vi "Node - Config Writer.vi"(8 "error in (no error)":errorcluster, 11 "Node Data In":T1) -> (0 "error out":errorcluster, 3 "Node Data Out":T1)   [LabVIEW 2016, in "PXImc Router.lvlib"]
uses:
  PXImc Router.lvlib
  Controls/Node Data.ctl
  <vilib>/NI Veristand/VeriStand Data/Byte Buffer/Byte Buffer.lvclass
  Controls/Node/Node - PXImc Parameters.ctl
  Controls/Node/Node - Writer Data.ctl
  Controls/Node/Node Ch Properties.ctl
  Controls/Data Type.ctl
  Controls/Node/Node - Readers Data.ctl
  Controls/Node/Node - Reader Data.ctl
  <vilib>/NI Veristand/VeriStand Data/Byte Buffer/Byte Buffer.lvclass/Byte Buffer.ctl
  <vilib>/NI Veristand/VeriStand Data/Byte Buffer/Byte Buffer.Get Buffer Pointer.vi
  <vilib>/NI Veristand/VeriStand Data/Byte Buffer/Byte Buffer.Get Buffer Size.vi
  <vilib>/NI Veristand/VeriStand Data/Memory Management/Memory Management.MoveByteBlock (Pointer).vi
  <vilib>/NI Veristand/VeriStand Data/Pointer Operations/Pointer.New.vi
  <vilib>/NI Veristand/VeriStand Data/Pointer Operations/Pointer.Dispose.vi
  <vilib>/NI Veristand/VeriStand Data/Byte Buffer/Byte Buffer.Set Buffer Pointer.vi
  <vilib>/NI Veristand/VeriStand Data/Byte Buffer/Byte Buffer.Set Buffer Size.vi
  <vilib>/NI Veristand/VeriStand Data/Memory Management/Memory Management.Handle Return.vi
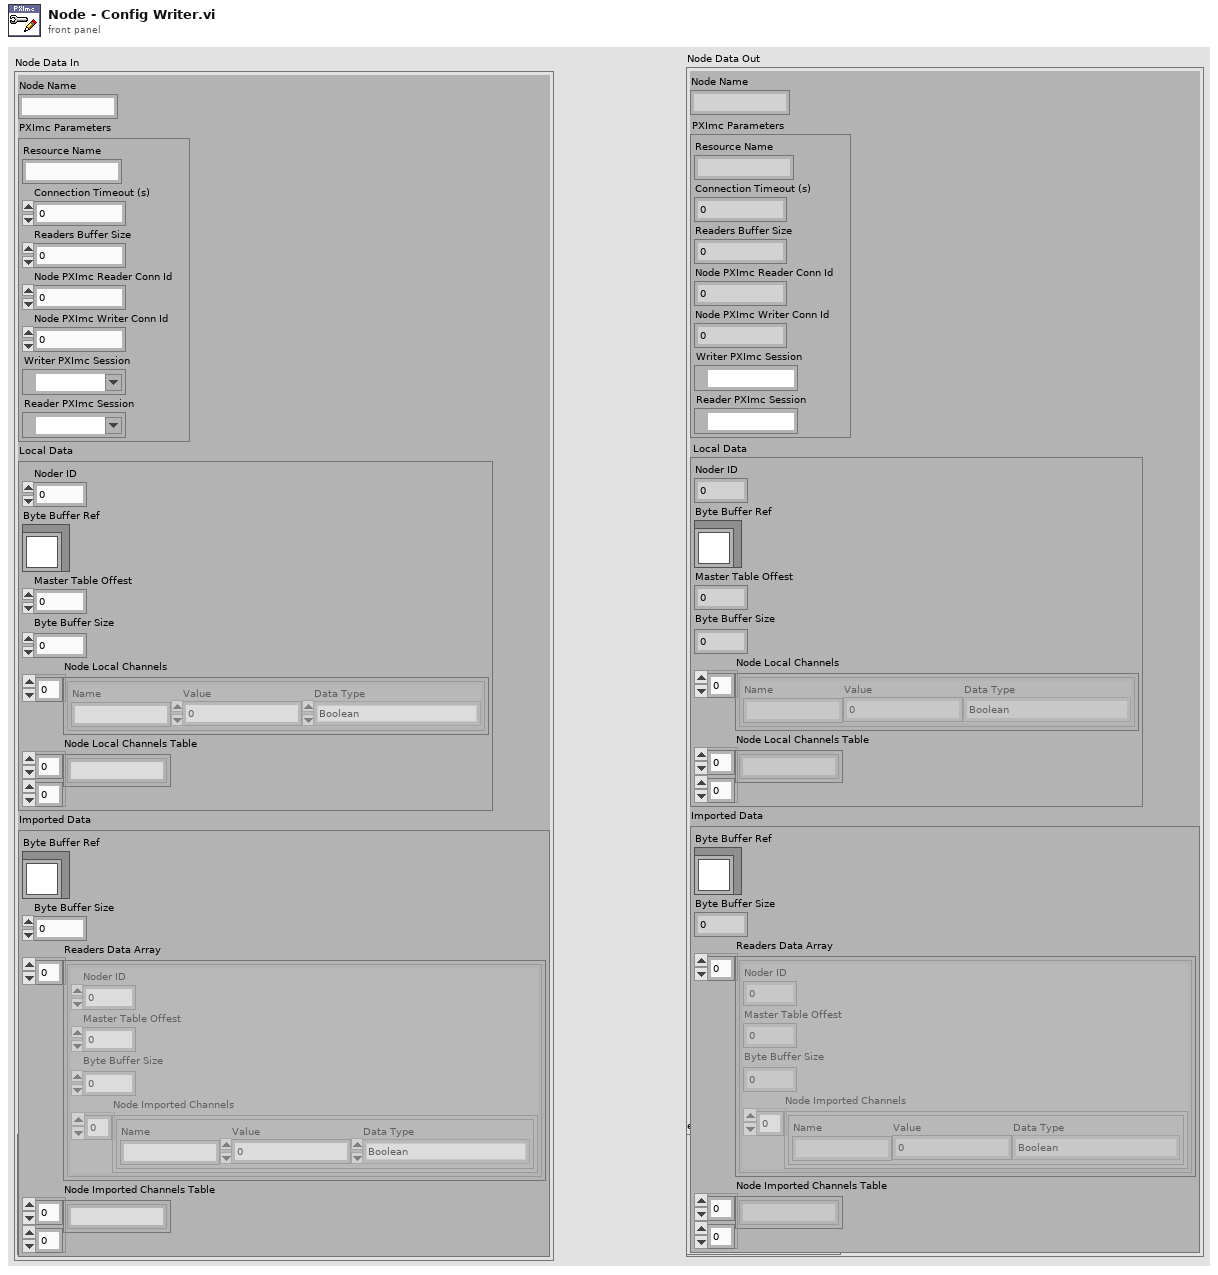
[diagram p1: front panel]
types:
  T1 = typedef "PXImc Router.lvlib/Node Data.ctl" = cluster{"Node Name":string, "PXImc Parameters":T2, "Local Data":T3, "Imported Data":T6}
  T2 = typedef "PXImc Router.lvlib/Node - PXImc Parameters.ctl" = cluster{"Resource Name":string, "Connection Timeout (s)":dbl, "Readers Buffer Size":u64, "Node PXImc Reader Conn Id":u16, "Node PXImc Writer Conn Id":u16, "Writer PXImc Session":refnum<k21>, "Reader PXImc Session":refnum<k21>}
  T3 = typedef "PXImc Router.lvlib/Node - Writer Data.ctl" = cluster{"Noder ID":u32, "Byte Buffer Ref":refnum<class "Byte Buffer.lvclass">, "Master Table Offest":u32, "Byte Buffer Size":u32, "Node Local Channels":T4[], "Node Local Channels Table":string[][]}
  T4 = typedef "PXImc Router.lvlib/Node Ch Properties.ctl" = cluster{"Name":string, "Value":dbl, "Data Type":T5}
  T5 = typedef "PXImc Router.lvlib/Data Type.ctl" = enum16{"Boolean", "SGL", "DBL", "I8", "I16", "I32", "I64", "U8", "U16", "U32", "U64"}
  T6 = typedef "PXImc Router.lvlib/Node - Readers Data.ctl" = cluster{"Byte Buffer Ref":refnum<class "Byte Buffer.lvclass">, "Byte Buffer Size":u64, "Readers Data Array":T7[], "Node Imported Channels Table":string[][]}
  T7 = typedef "PXImc Router.lvlib/Node - Reader Data.ctl" = cluster{"Noder ID":u32, "Master Table Offest":u32, "Byte Buffer Size":u64, "Node Imported Channels":T4[]}
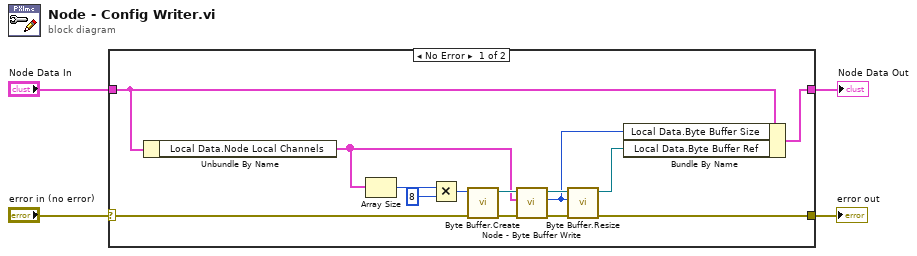
[diagram p0: block diagram]
diagram:
  n1 = case shown="No Error" "error in (no error)" {
    selector: "error in (no error)" -> [w6 w20]
    tunnel: [w18 w20] -> w4
    tunnel: [w8 w19] -> w3
    tunnel: "Node Data In" -> [w7 w19]
    frame No Error {
      n2 = Unbundle By Name(w7) -> ("Local Data.Node Local Channels"=w5:T4[])
      n3 = Array Size(array=w5) -> (size(s)=w15:i32)
      n4 = Multiply(x=w15, y=8) -> (x*y=w13:i32)
      n5 = call <vilib>:"Byte Buffer.Create.vi"("error in (no error)"=w6, "size"=w13) -> ("error out"=w16:errorcluster, "Byte Buffer"=w17:refnum<class "Byte Buffer.lvclass">)  [unwired: 8 in]
      n6 = call "Node - Byte Buffer Write.vi"("error in (no error)"=w16, "Node Local Channels"=w5, "Byte Buffer In"=w17) -> ("error out"=w11:errorcluster, "Buffer Offset Out"=w9:u64, "Byte Buffer Out"=w12:refnum<class "Byte Buffer.lvclass">)  [unwired: 5 in, 1 out]
      n7 = call <vilib>:"Byte Buffer.Resize.vi"("error in (no error)"=w11, "new size"=w9, "Byte Buffer in"=w12) -> ("error out"=w18:errorcluster, "Byte Buffer out"=w10:refnum<class "Byte Buffer.lvclass">)  [unwired: 7 in]
      n8 = Bundle By Name(cluster=w7, "Local Data.Byte Buffer Size"=w9, "Local Data.Byte Buffer Ref"=w10) -> (w8:T1)
    }
    frame Error {
    }
  }
  "error out" <- w4
  "Node Data Out" <- w3
